vi "filesave.vi"(0 "Temperature\nInput":dbl, 1 "Counter\nInput":dbl) -> ()   [LabVIEW 2023]
uses:
  <vilib>/express/express shared/transition.llb/Dynamic To Waveform Array.vi
  <vilib>/express/express signal manip/GetorSetDDTAttributes/Set DDT Attributes/SetT0.vi
  <vilib>/express/express shared/transition.llb/Waveform Array To Dynamic.vi
  <vilib>/express/express signal manip/GetorSetDDTAttributes/Set DDT Attributes/Set DDT Properties.xnode
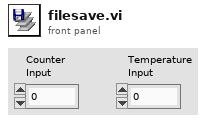
[diagram p1: front panel]
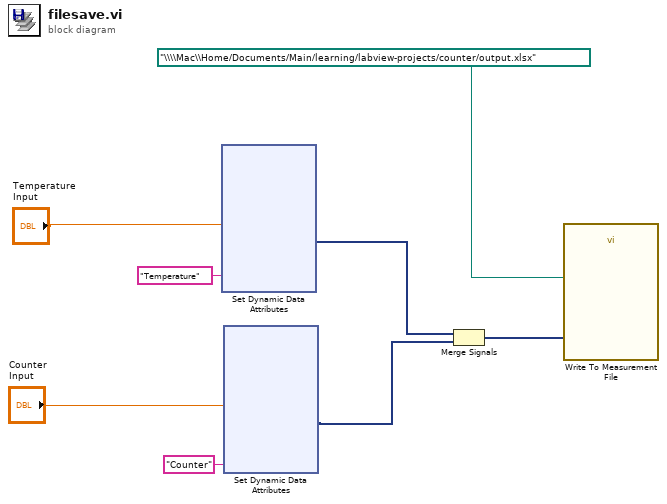
[diagram p0: block diagram]
diagram:
  n1 = xnode "Set Dynamic Data Attributes"("Signals In"="Temperature\nInput", "Signal Name"="Temperature") -> ("Signals Out"=w3:dynamicdata)  [unwired: 2 in, 1 out]
  n2 = xnode "Set Dynamic Data Attributes"("Signals In"="Counter\nInput", "Signal Name"="Counter") -> ("Signals Out"=w1:dynamicdata)  [unwired: 2 in, 1 out]
  n3 = Merge Signals(w3, w1) -> (w8:dynamicdata)
  n4 = call "Write To Measurement File"("Signals"=w8, "Filename"=path "\\\\Mac\\Home/Documents/Main/learning/labview-projects/counter/output.xlsx") -> ()  [unwired: 15 in, 3 out]
